vi "DataVIS_Read Entire .DAT Data.vi"(8 "error in (no error)":errorcluster, 11 "file path (use dialog)":path) -> (0 "error out":errorcluster, 3 "data value reference":refnum<data-value>)   [LabVIEW 2016]
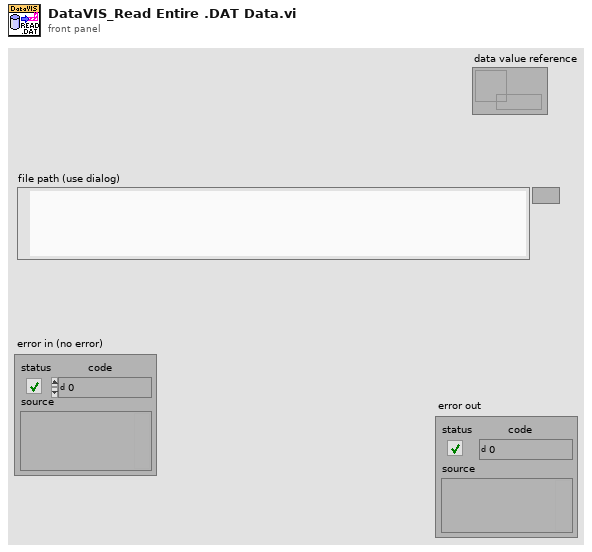
[diagram p1: front panel]
types:
  T1 = enum16{"open", "replace", "create", "open or create", "replace or create", "replace or create with confirmation"}
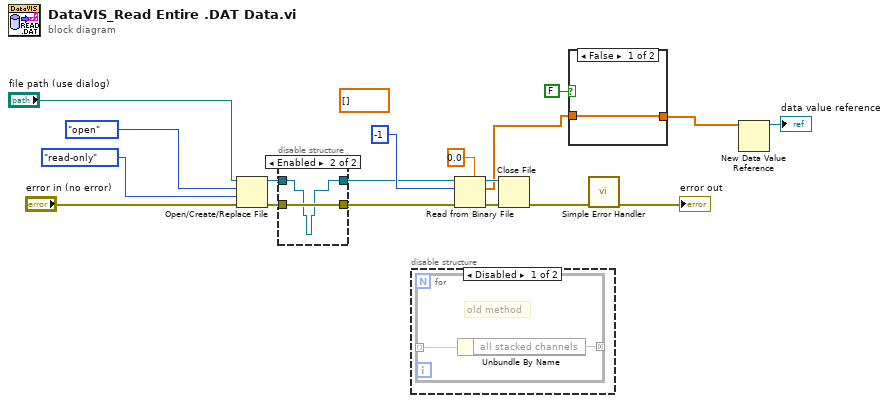
[diagram p0: block diagram]
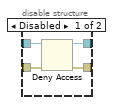
[diagram p4: hidden frame]
diagram:
  (unwired) dbl[] [] ("all stacked channels")
  n1 = Open/Create/Replace File(file path (use dialog)="file path (use dialog)", error in="error in (no error)", operation (0:open)=T1."open", access (0:read/write)=enum16{"read/write", "read-only", "write-only"}."read-only") -> (refnum out=w6:refnum<file>, error out=w15:errorcluster)  [unwired: 2 in, 1 out]
  n2 = disable-structure shown="Enabled" {
    disable-tunnel: w6 -> [w22 w23]
    disable-tunnel: w15 -> [w21 w24]
    disable-tunnel: [w20 w24] -> w8
    disable-tunnel: [w19 w23] -> w7
    frame Disabled {
      n3 = Deny Access(4:w21, 7:w22) -> (0:w20:errorcluster, 3:w19:refnum<file>)  [unwired: 1 in]
    }
    frame Enabled {
    }
  }
  n4 = disable-structure shown="Disabled" {
    frame Disabled {
      n5 = for {
        tunnel: _ -> [w26] mode=indexing
        tunnel: [w25] -> _ mode=concatenating
        # "old method"
        n6 = Unbundle By Name(w26) -> ("all stacked channels"=w25)
      }
    }
    frame Enabled {
    }
  }
  n7 = Read from Binary File(5:0.0, 8:w8, 10:-1 ("count (1)"), 11:w7) -> (0:w12:errorcluster, 2:w3:dbl[], 3:w11:refnum<file>)  [unwired: 2 in, 1 out]
  n8 = Close File(refnum=w11, error in=w12) -> (error out=w13:errorcluster)  [unwired: 1 out]
  n9 = case shown="False" FALSE {
    tunnel: w3 -> [w27 w28]
    tunnel: [w27 w28] -> w2
    frame False {
    }
    frame True {
    }
  }
  n10 = call <vilib>:"Simple Error Handler.vi"("error in (no error)"=w13) -> ("error out"=→"error out":errorcluster)  [unwired: 4 in, 4 out]
  n11 = New Data Value Reference(data value=w2) -> (data value reference=→"data value reference":refnum<data-value>)  [unwired: 1 in, 1 out]
